vi "HSV to RGB.vi"(0 "Hue":dbl, 5 "Saturation":dbl=1.0, 7 "Value":dbl, 11 "error in":errorcluster) -> (4 "Color":u32(colorbox), 15 "error out":errorcluster)   [LabVIEW 2015, in "niHighSpeedSerial Eye Scan v1 Host.lvclass"]
uses:
  <instrlib>/niHighSpeedSerial/Eye Scan/v1/Host/Eye Scan/niHighSpeedSerial Eye Scan v1 Host.lvclass
panel:
  out "Red":u8
  out "Green":u8
  out "Blue":u8
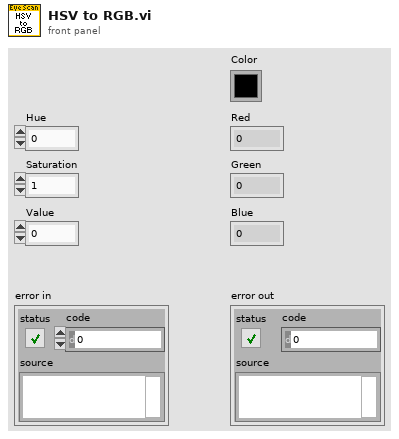
[diagram p1: front panel]
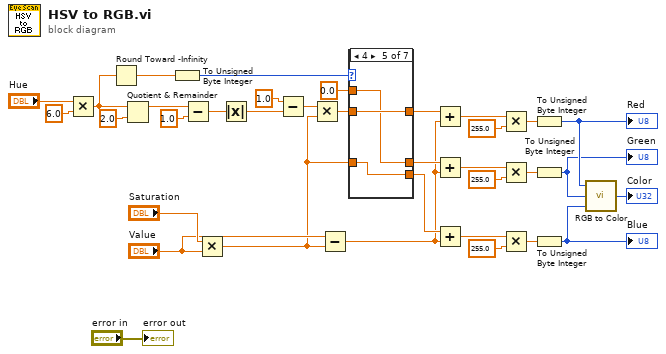
[diagram p0: block diagram]
diagram:
  n1 = Multiply(x="Hue", y=6.0) -> (x*y=w13:dbl)
  n2 = Round Toward -Infinity(1:w13) -> (0:w31:dbl)
  n3 = Quotient & Remainder(x=w13, y=2.0) -> (x-y*floor(x/y)=w11:dbl)  [unwired: 1 out]
  n4 = To Unsigned Byte Integer(number=w31) -> (unsigned 8bit integer=w14:u8)
  n5 = Subtract(x=w11, y=1.0) -> (x-y=w9:dbl)
  n6 = Multiply(x="Saturation", y="Value") -> (x*y=w28:dbl)
  n7 = Absolute Value(x=w9) -> (abs(x)=w8:dbl)
  n8 = Subtract(x=1.0, y=w8) -> (x-y=w6:dbl)
  n9 = Multiply(x=w6, y=w28) -> (x*y=w30:dbl)
  n10 = Subtract(x="Value", y=w28) -> (x-y=w24:dbl)
  n11 = case shown="4" w14 {
    tunnel: w28 -> [w38 w40 w43 w45 w48 w53 _]
    tunnel: w30 -> [w37 w41 w42 w46 w50 w51 _]
    tunnel: 0.0 -> [w36 w39 w44 w47 w49 w52 w54]
    tunnel: [w38 w41 w44 w47 w50 w53 w54] -> w25
    tunnel: [w37 w40 w43 w46 w49 w52 w54] -> w26
    tunnel: [w36 w39 w42 w45 w48 w51 w54] -> w27
    frame 0 {
    }
    frame 1 {
    }
    frame 2 {
    }
    frame 3 {
    }
    frame 4 {
    }
    frame 5 {
    }
    frame Default {
    }
  }
  n12 = Add(x=w25, y=w24) -> (x+y=w15:dbl)
  n13 = Add(x=w26, y=w24) -> (x+y=w16:dbl)
  n14 = Add(x=w27, y=w24) -> (x+y=w17:dbl)
  n15 = Multiply(x=w15, y=255.0) -> (x*y=w22:dbl)
  n16 = Multiply(x=w16, y=255.0) -> (x*y=w21:dbl)
  n17 = Multiply(x=w17, y=255.0) -> (x*y=w19:dbl)
  n18 = To Unsigned Byte Integer(number=w22) -> (unsigned 8bit integer=w5:u8)
  "Red" <- w5
  n19 = To Unsigned Byte Integer(number=w21) -> (unsigned 8bit integer=w4:u8)
  "Green" <- w4
  n20 = To Unsigned Byte Integer(number=w19) -> (unsigned 8bit integer=w3:u8)
  "Blue" <- w3
  n21 = call <vilib>:"RGB to Color.vi"("B"=w3, "G"=w4, "R"=w5) -> ("Color"=→"Color":u32)
  "error out" <- "error in"
